vi "R1Initialize.vi"(8 "error in (no error)":errorcluster) -> (0 "error out":errorcluster)   [LabVIEW 2016]
uses:
  Controls/R1SBR_SetParams.ctl
  Controls/pH_SetParams Standard.ctl
  Controls/pH_Manual Standard.ctl
  Controls/ISE_CF.ctl
panel:
  out "?":dbl
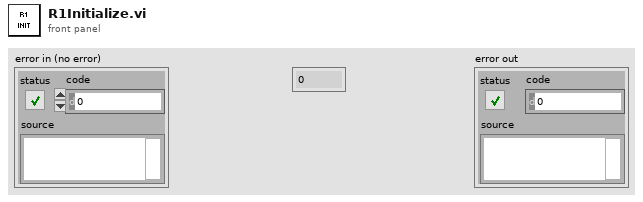
[diagram p1: front panel]
types:
  T1 = cluster{"Set Point, mgN/L":dbl, "Tolerance, mgN/L":dbl, "Pump Gain":dbl, "Max Volume/Cycle, mL":dbl}
  T2 = typedef "ISE_CF.ctl" = cluster{"Correction Factor":dbl, "Ion":string, "Correct For Ion?":bool}
  T3 = cluster{"Equil Approach Set point, mV/min":dbl, "Equil Approach dt, s":dbl, "Interference Correction Factors":T2[], "Detect Equilibrium?":bool, "Probe Intercept":dbl, "Probe Slope":dbl, "Baseline":dbl, "Detection Limit, M":dbl}
  T4 = cluster{"Media Pump":bool, "Water Pump":bool, "Effluent Pump":bool, "Release Valve":bool, "Gas Pump":bool}
  T5 = cluster{"Set Point, mg/L":dbl, "Tolerance, mg/L":dbl, "N2 Valve Gain":dbl, "Air Valve Gain":dbl}
  T6 = typedef "pH_SetParams Standard.ctl" = cluster{"Set Point":dbl, "Tolerance":dbl, "Pump Time On, secs":dbl}
  T7 = typedef "R1SBR_SetParams.ctl" = cluster{"Phase":string, "Time, min":dbl, "SBR_Manual":cluster{"Media Pump":bool, "Water Pump":bool, "Effluent Pump":bool, "Release Valve":bool, "Gas Pump":bool}}[]
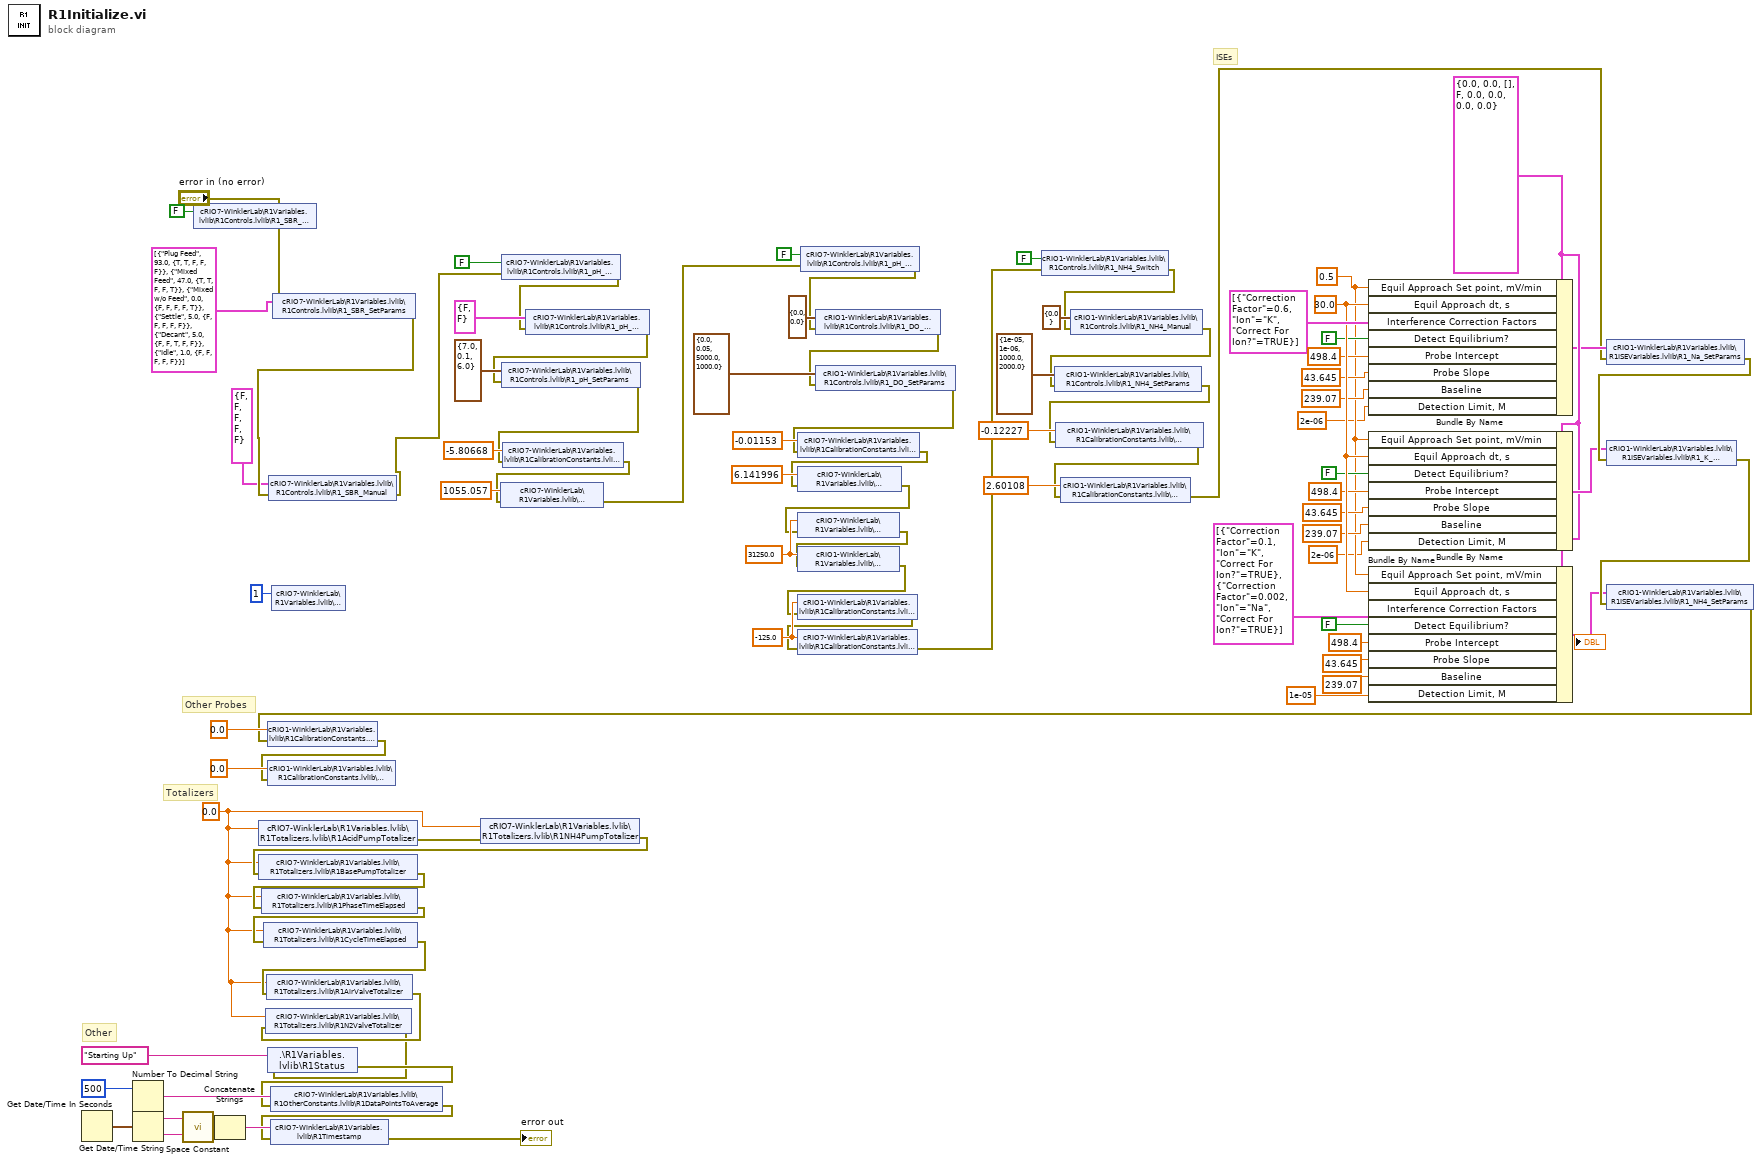
[diagram p0: block diagram]
diagram:
  w22 = T3 {"Equil Approach Set point, mV/min"=0.0, "Equil Approach dt, s"=0.0, "Interference Correction Factors"=[], "Detect Equilibrium?"=FALSE, "Probe Intercept"=0.0, "Probe Slope"=0.0, "Baseline"=0.0, "Detection Limit, M"=0.0} ("R1NaSetParams")
  w42 = 30.0 ("Equil Approach dt, s")
  w23 = 0.5 ("Equil Approach Set point, mV/min")
  w1 = 0.0 ("R1PhaseTimeElapsed")
  w76 = 31250.0 ("R1AirSlope")
  w77 = -125.0 ("R1N2Intercept")
  # "ISEs"
  # "Totalizers"
  # "Other Probes"
  # "Other"
  n1 = Get Date/Time In Seconds() -> (seconds since 1Jan1904=w55:timestamp)
  n2 = Number To Decimal String(number=500 ("R1DataPointsToAverage")) -> (decimal integer string=w82:string)  [unwired: 1 in]
  n3 = Get Date/Time String(seconds (now)=w55) -> (date string=w48:string, time string=w54:string)  [unwired: 2 in]
  n4 = call <vilib>:"Space Constant.vi"() -> ("String"=w53:string)
  n5 = shared-variable "cRIO7-WinklerLab\\R1Variables.lvlib\\R1Controls.lvlib\\R1_SBR_Switch"(FALSE ("R1SBRSwitch")) -> ()  [unwired: 1 in, 1 out]
  n6 = Concatenate Strings(w48, w53, w54) -> (w51:string)
  n7 = shared-variable "cRIO7-WinklerLab\\R1Variables.lvlib\\R1Totalizers.lvlib\\R1AcidPumpTotalizer"(w1) -> (error out=w5:errorcluster)  [unwired: 1 in]
  n8 = shared-variable "cRIO7-WinklerLab\\R1Variables.lvlib\\R1OtherConstants.lvlib\\R1No"(i16 1 ("R1No")) -> ()  [unwired: 1 in, 1 out]
  n9 = shared-variable "cRIO7-WinklerLab\\R1Variables.lvlib\\R1Controls.lvlib\\R1_SBR_SetParams"(T7 [{"Phase"="Plug Feed", "Time, min"=93.0, "SBR_Manual"={"Media Pump"=TRUE, "Water Pump"=TRUE, "Effluent Pump"=FALSE, "Release Valve"=FALSE, "Gas Pump"=FALSE}}, {"Phase"="Mixed Feed", "Time, min"=47.0, "SBR_Manual"={"Media Pump"=TRUE, "Water Pump"=TRUE, "Effluent Pump"=FALSE, "Release Valve"=FALSE, "Gas Pump"=TRUE}}, {"Phase"="Mixed w/o Feed", "Time, min"=0.0, "SBR_Manual"={"Media Pump"=FALSE, "Water Pump"=FALSE, "Effluent Pump"=FALSE, "Release Valve"=FALSE, "Gas Pump"=TRUE}}, {"Phase"="Settle", "Time, min"=5.0, "SBR_Manual"={"Media Pump"=FALSE, "Water Pump"=FALSE, "Effluent Pump"=FALSE, "Release Valve"=FALSE, "Gas Pump"=FALSE}}, {"Phase"="Decant", "Time, min"=5.0, "SBR_Manual"={"Media Pump"=FALSE, "Water Pump"=FALSE, "Effluent Pump"=TRUE, "Release Valve"=FALSE, "Gas Pump"=FALSE}}, {"Phase"="Idle", "Time, min"=1.0, "SBR_Manual"={"Media Pump"=FALSE, "Water Pump"=FALSE, "Effluent Pump"=FALSE, "Release Valve"=FALSE, "Gas Pump"=FALSE}}] ("R1SBR_SetParams 2"), error in="error in (no error)") -> (error out=w46:errorcluster)
  n10 = shared-variable "cRIO7-WinklerLab\\R1Variables.lvlib\\R1Controls.lvlib\\R1_SBR_Manual"(T4 {"Media Pump"=FALSE, "Water Pump"=FALSE, "Effluent Pump"=FALSE, "Release Valve"=FALSE, "Gas Pump"=FALSE} ("R1SBRManual"), error in=w46) -> (error out=w44:errorcluster)
  n11 = shared-variable "cRIO7-WinklerLab\\R1Variables.lvlib\\R1Totalizers.lvlib\\R1NH4PumpTotalizer"(w1, error in=w5) -> (error out=w6:errorcluster)
  n12 = shared-variable "cRIO7-WinklerLab\\R1Variables.lvlib\\R1Totalizers.lvlib\\R1BasePumpTotalizer"(w1, error in=w6) -> (error out=w49:errorcluster)
  n13 = shared-variable "cRIO7-WinklerLab\\R1Variables.lvlib\\R1Totalizers.lvlib\\R1PhaseTimeElapsed"(w1, error in=w49) -> (error out=w56:errorcluster)
  n14 = shared-variable "cRIO7-WinklerLab\\R1Variables.lvlib\\R1Totalizers.lvlib\\R1CycleTimeElapsed"(w1, error in=w56) -> (error out=w4:errorcluster)
  n15 = shared-variable "cRIO7-WinklerLab\\R1Variables.lvlib\\R1Totalizers.lvlib\\R1AirValveTotalizer"(w1, error in=w4) -> (error out=w3:errorcluster)
  n16 = shared-variable "cRIO7-WinklerLab\\R1Variables.lvlib\\R1Totalizers.lvlib\\R1N2ValveTotalizer"(w1, error in=w3) -> (error out=w2:errorcluster)
  n17 = shared-variable ".\\R1Variables.lvlib\\R1Status"("Starting Up" ("R1Status"), error in=w2) -> (error out=w58:errorcluster)
  n18 = shared-variable "cRIO7-WinklerLab\\R1Variables.lvlib\\R1OtherConstants.lvlib\\R1DataPointsToAverage"(w82, error in=w58) -> (error out=w50:errorcluster)
  n19 = shared-variable "cRIO7-WinklerLab\\R1Variables.lvlib\\R1Timestamp"(w51, error in=w50) -> (error out=→"error out":errorcluster)
  n20 = shared-variable "cRIO7-WinklerLab\\R1Variables.lvlib\\R1Controls.lvlib\\R1_pH_Switch"(FALSE ("R1pHSwitch"), error in=w44) -> (error out=w72:errorcluster)
  n21 = shared-variable "cRIO7-WinklerLab\\R1Variables.lvlib\\R1Controls.lvlib\\R1_pH_Manual"(cluster{"Acid Pump":bool, "Base Pump":bool} {"Acid Pump"=FALSE, "Base Pump"=FALSE} ("R1pHManual"), error in=w72) -> (error out=w71:errorcluster)
  n22 = shared-variable "cRIO7-WinklerLab\\R1Variables.lvlib\\R1Controls.lvlib\\R1_pH_SetParams"(T6 {"Set Point"=7.0, "Tolerance"=0.1, "Pump Time On, secs"=6.0} ("R1pHSetParams"), error in=w71) -> (error out=w70:errorcluster)
  n23 = shared-variable "cRIO7-WinklerLab\\R1Variables.lvlib\\R1CalibrationConstants.lvlib\\R1pHIntercept"(-5.80668 ("R12pHInt"), error in=w70) -> (error out=w67:errorcluster)
  n24 = shared-variable "cRIO7-WinklerLab\\R1Variables.lvlib\\R1CalibrationConstants.lvlib\\R1pHSlope"(1055.057 ("R1pHSlope"), error in=w67) -> (error out=w68:errorcluster)
  n25 = shared-variable "cRIO7-WinklerLab\\R1Variables.lvlib\\R1Controls.lvlib\\R1_pH_Switch"(FALSE ("R1pHSwitch"), error in=w68) -> (error out=w66:errorcluster)
  n26 = shared-variable "cRIO1-WinklerLab\\R1Variables.lvlib\\R1Controls.lvlib\\R1_DO_Manual"(cluster{"Air MFC":dbl, "N2 MFC":dbl} {"Air MFC"=0.0, "N2 MFC"=0.0} ("R1DOManual"), error in=w66) -> (error out=w65:errorcluster)
  n27 = shared-variable "cRIO1-WinklerLab\\R1Variables.lvlib\\R1Controls.lvlib\\R1_DO_SetParams"(T5 {"Set Point, mg/L"=0.0, "Tolerance, mg/L"=0.05, "N2 Valve Gain"=5000.0, "Air Valve Gain"=1000.0} ("R1DOSetParams"), error in=w65) -> (error out=w64:errorcluster)
  n28 = shared-variable "cRIO7-WinklerLab\\R1Variables.lvlib\\R1CalibrationConstants.lvlib\\R1DOIntercept"(-0.01153 ("R1DOInt"), error in=w64) -> (error out=w63:errorcluster)
  n29 = shared-variable "cRIO7-WinklerLab\\R1Variables.lvlib\\R1CalibrationConstants.lvlib\\R1DOSlope"(6.141996 ("R1DOSlope"), error in=w63) -> (error out=w62:errorcluster)
  n30 = shared-variable "cRIO7-WinklerLab\\R1Variables.lvlib\\R1CalibrationConstants.lvlib\\R1N2Slope"(w76, error in=w62) -> (error out=w61:errorcluster)
  n31 = shared-variable "cRIO1-WinklerLab\\R1Variables.lvlib\\R1CalibrationConstants.lvlib\\R1AirSlope"(w76, error in=w61) -> (error out=w60:errorcluster)
  n32 = shared-variable "cRIO1-WinklerLab\\R1Variables.lvlib\\R1CalibrationConstants.lvlib\\R1AirIntercept"(w77, error in=w60) -> (error out=w59:errorcluster)
  n33 = shared-variable "cRIO7-WinklerLab\\R1Variables.lvlib\\R1CalibrationConstants.lvlib\\R1N2Intercept"(w77, error in=w59) -> (error out=w12:errorcluster)
  n34 = shared-variable "cRIO1-WinklerLab\\R1Variables.lvlib\\R1Controls.lvlib\\R1_NH4_Switch"(FALSE ("R1_NH4_Switch"), error in=w12) -> (error out=w11:errorcluster)
  n35 = shared-variable "cRIO1-WinklerLab\\R1Variables.lvlib\\R1Controls.lvlib\\R1_NH4_Manual"(cluster{"NH4 Pump Flowrate, ml/min":dbl} {"NH4 Pump Flowrate, ml/min"=0.0} ("R1NH4Manual"), error in=w11) -> (error out=w10:errorcluster)
  n36 = shared-variable "cRIO1-WinklerLab\\R1Variables.lvlib\\R1Controls.lvlib\\R1_NH4_SetParams"(T1 {"Set Point, mgN/L"=1e-05, "Tolerance, mgN/L"=1e-06, "Pump Gain"=1000.0, "Max Volume/Cycle, mL"=2000.0} ("R1_NH4_SetParams"), error in=w10) -> (error out=w9:errorcluster)
  n37 = shared-variable "cRIO1-WinklerLab\\R1Variables.lvlib\\R1CalibrationConstants.lvlib\\NH4PumpIntercept"(-0.12227 ("NH4PumpIntercept"), error in=w9) -> (error out=w8:errorcluster)
  n38 = shared-variable "cRIO1-WinklerLab\\R1Variables.lvlib\\R1CalibrationConstants.lvlib\\NH4PumpSlope"(2.60108 ("NH4PumpSlope"), error in=w8) -> (error out=w7:errorcluster)
  n39 = Bundle By Name(cluster=w22, "Equil Approach Set point, mV/min"=w23, "Equil Approach dt, s"=w42, "Interference Correction Factors"=T2[] [{"Correction Factor"=0.6, "Ion"="K", "Correct For Ion?"=TRUE}], "Detect Equilibrium?"=FALSE, "Probe Intercept"=498.4, "Probe Slope"=43.645 ("Equil Approach dt, s"), "Baseline"=239.07 ("Equil Approach dt, s"), "Detection Limit, M"=2e-06) -> (w19:T3)
  n40 = Bundle By Name(cluster=w22, "Equil Approach Set point, mV/min"=w23, "Equil Approach dt, s"=w42, "Detect Equilibrium?"=FALSE, "Probe Intercept"=498.4, "Probe Slope"=43.645 ("Equil Approach dt, s"), "Baseline"=239.07 ("Equil Approach dt, s"), "Detection Limit, M"=2e-06) -> (w37:T3)
  n41 = Bundle By Name(cluster=w22, "Equil Approach Set point, mV/min"=w23, "Equil Approach dt, s"=w42, "Interference Correction Factors"=T2[] [{"Correction Factor"=0.1, "Ion"="K", "Correct For Ion?"=TRUE}, {"Correction Factor"=0.002, "Ion"="Na", "Correct For Ion?"=TRUE}], "Detect Equilibrium?"=FALSE, "Probe Intercept"=498.4, "Probe Slope"=43.645 ("Equil Approach dt, s"), "Baseline"=239.07 ("Equil Approach dt, s"), "Detection Limit, M"=1e-05) -> (w36:T3)
  n42 = shared-variable "cRIO1-WinklerLab\\R1Variables.lvlib\\R1ISEVariables.lvlib\\R1_Na_SetParams"(w19, error in=w7) -> (error out=w40:errorcluster)
  n43 = shared-variable "cRIO1-WinklerLab\\R1Variables.lvlib\\R1ISEVariables.lvlib\\R1_K_SetParams"(w37, error in=w40) -> (error out=w39:errorcluster)
  n44 = shared-variable "cRIO1-WinklerLab\\R1Variables.lvlib\\R1ISEVariables.lvlib\\R1_NH4_SetParams"(w36, error in=w39) -> (error out=w38:errorcluster)
  n45 = shared-variable "cRIO1-WinklerLab\\R1Variables.lvlib\\R1CalibrationConstants.lvlib\\R1ORPSlope"(0.0 ("R1ORPSlope"), error in=w38) -> (error out=w57:errorcluster)
  n46 = shared-variable "cRIO1-WinklerLab\\R1Variables.lvlib\\R1CalibrationConstants.lvlib\\R1ORPIntercept"(0.0 ("R1ORPIntercept"), error in=w57) -> ()  [unwired: 1 out]
